vi "Timeout.vi"(2 "Start Time In":u32, 3 "Limit In":u32) -> (0 "Start Time Out":u32, 1 "Timeout":bool=TRUE)   [LabVIEW 2013]
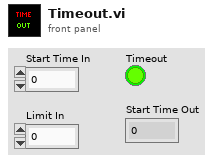
[diagram p1: front panel]
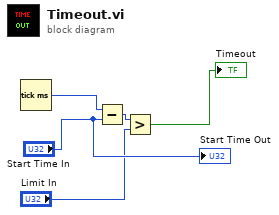
[diagram p0: block diagram]
diagram:
  n1 = Tick Count (ms)() -> (millisecond timer value=w1:u32)
  n2 = Subtract(x=w1, y="Start Time In") -> (x-y=w2:u32)
  n3 = Greater?(x=w2, y="Limit In") -> (0:→"Timeout":bool)
  "Start Time Out" <- "Start Time In"
